vi "读取查询间隔.vi"(8 "error in (no error)":errorcluster caption="错误输入（无错误）", 11 "客户端输入":refnum<class "客户端.lvclass">) -> (0 "error out":errorcluster caption="错误输出", 2 "查询间隔":i32, 3 "客户端输出":refnum<class "客户端.lvclass">)   [LabVIEW 2015, in "客户端.lvlib" / "客户端.lvclass"]
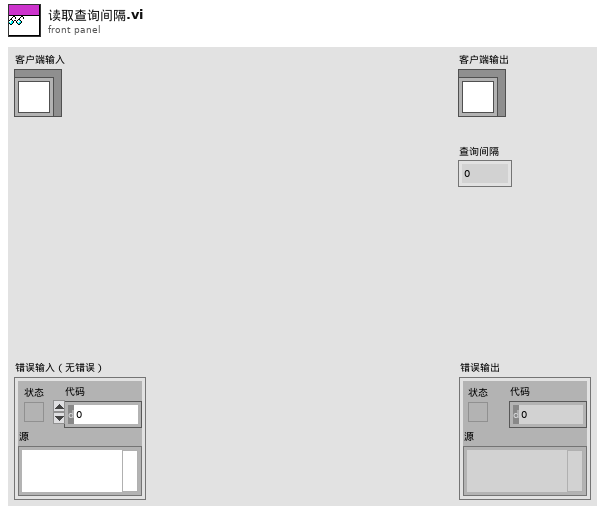
[diagram p1: front panel]
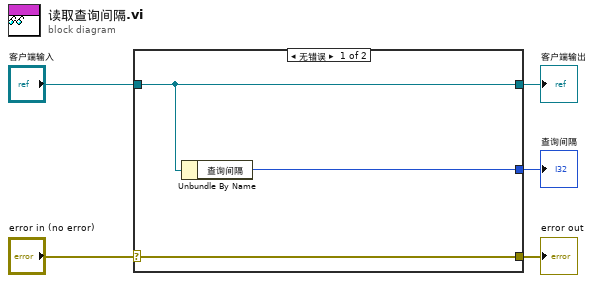
[diagram p0: block diagram]
diagram:
  n1 = case shown="无错误" "error in (no error)" {
    selector: "error in (no error)" -> [w8 w9]
    tunnel: [w8 w9] -> w4
    tunnel: [w7 w10] -> w2
    tunnel: "客户端输入" -> [w7 w10]
    tunnel: [w6 _] -> w1
    frame No Error {
      n2 = Unbundle By Name(w7) -> ("查询间隔"=w6:i32)
    }
    frame Error {
    }
  }
  "error out" <- w4
  "客户端输出" <- w2
  "查询间隔" <- w1
